vi "Voltage_Continuous_Output-Clear_data_when_stop.vi"() -> ()   [LabVIEW 2018]
doc: "This example demonstrates how to continuously re-generate analog output data from a buffer in your computer's memory.\n\nRefer to your device documentation for pinouts and hardware capabilities."
uses:
  <vilib>/Utility/error.llb/DialogType.ctl
  <vilib>/DAQmx/write.llb/DAQmx Write (Analog 1D Wfm NChan NSamp).vi
  <vilib>/DAQmx/create/channels.llb/DAQmx Create Channel (AO-Voltage-Basic).vi
  <vilib>/DAQmx/configure/timing.llb/DAQmx Timing (Sample Clock).vi
  <vilib>/DAQmx/miscellaneous.llb/DAQmx Fill In Error Info.vi
  <resource>/objmgr/daqmx.rc
  <vilib>/measure/NI_MABase.lvlib
panel:
  in  "Number of Samples":i32=1000
  in  "Output Array":T1(array[cluster])=[{"Waveform Type"=0, "Amplitude"=1.0, "Frequency"=10.0}] {"Frequency" format="%0.2p"; "Amplitude" format="%0.2p"; "Waveform Type" items=["Sine Wave", "Triangle Wave", "Square Wave", "Sawtooth Wave"]}
  in  "Stop":bool
  out "Waveform Graph":waveform(dbl)[](graph)=[{"t0"=timestamp(0 s since 1904-01-01), "dt"=0.001, "Y"=[]}]
  in  "Sample Rate":dbl=1000.0
  in  "Max Voltage":dbl=5.0
  in  "Min Voltage":dbl=-5.0
  in  "Physical Channel(s)":tag="Dev1/ao0"
  out "Actual Sample Rate":dbl=1000.0 format="%0.2f"
  # "Channel Settings"
  # "Output"
  # "Waveform Settings"
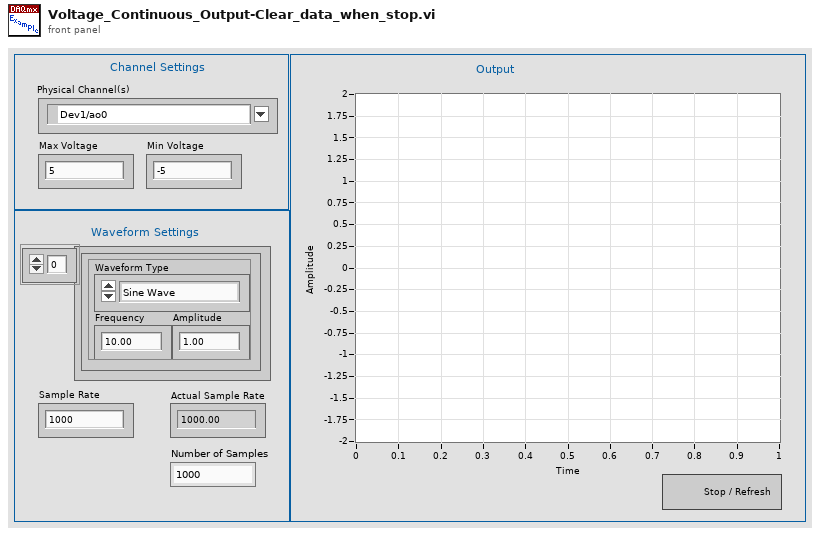
[diagram p1: front panel]
types:
  T1 = cluster{"Waveform Type":u16, "Amplitude":dbl, "Frequency":dbl}[]
  T2 = typedef "DialogType.ctl" = u16
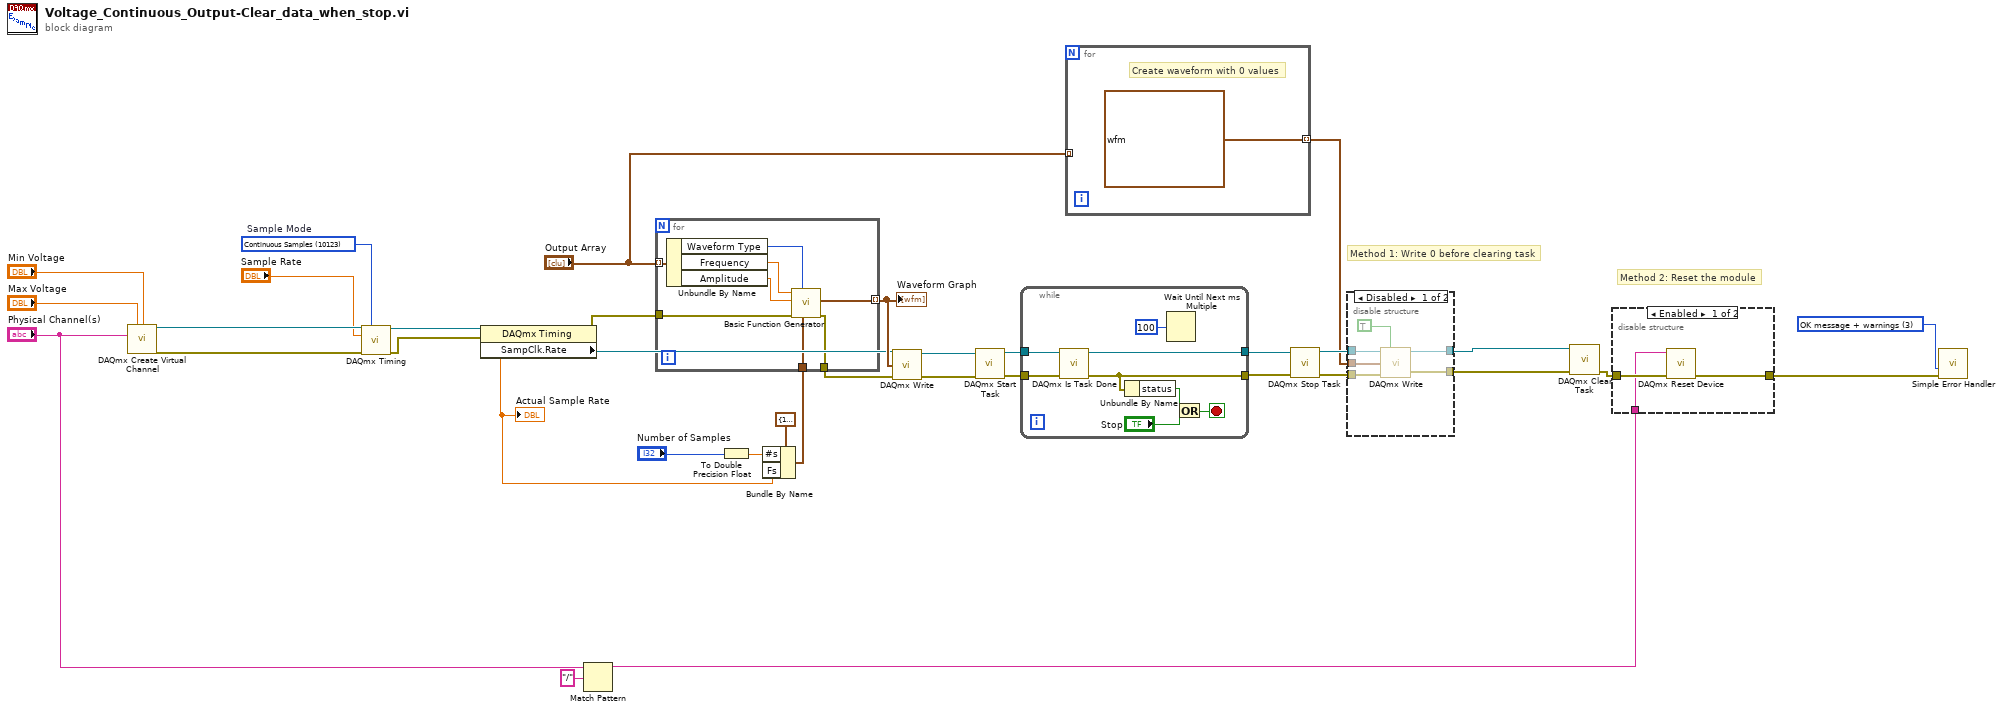
[diagram p0: block diagram]
diagram:
  w19 = T2 3 items=["no dialog", "OK message", "continue or stop message", "OK message + warnings", "continue/stop + warnings"] ("type of dialog (OK msg:1)")
  w33 = 10123 items=["Finite Samples"=10178, "Continuous Samples"=10123, "Hardware Timed Single Point"=12522]  # Sample Mode
  # "Method 2: Reset the module"
  # "Method 1: Write 0 before clearing task"
  n1 = call-poly <vilib>:"DAQmx Create Virtual Channel.vi"("maximum value"="Max Voltage", "minimum value"="Min Voltage", "physical channels"="Physical Channel(s)") -> ("task out"=w31:refnum<k21>, "error out"=w32:errorcluster)  [unwired: 11 in]
  n2 = call-poly <vilib>:"DAQmx Timing.vi"("task/channels in"=w31, "sample mode"=w33, "rate"="Sample Rate", "error in"=w32) -> ("task out"=w35:refnum<k21>, "error out"=w34:errorcluster)  [unwired: 10 in]
  n3 = property class="DAQmx Timing"(reference=w35, error in=w34) -> (reference out=w18:refnum<k21>, error out=w17:errorcluster, "SampClk.Rate"=w2:dbl)
  "Actual Sample Rate" <- w2
  n4 = Match Pattern(string="Physical Channel(s)", regular expression="/") -> (before substring=w12:string)  [unwired: 1 in, 3 out]
  n5 = To Double Precision Float(number="Number of Samples") -> (double precision float=w4:dbl)
  n6 = Bundle By Name(cluster=cluster{"Fs":dbl, "#s":dbl} {"Fs"=1000.0, "#s"=1000.0} ("sampling info"), "#s"=w4, "Fs"=w2) -> (w1:cluster{"Fs":dbl, "#s":dbl})
  n7 = for {
    tunnel: w17 -> [w43]
    tunnel: [w42] -> w23
    tunnel: "Output Array" -> [w41] mode=indexing
    tunnel: [w37] -> w22 mode=indexing
    tunnel: w1 -> [w36]
    n8 = Unbundle By Name(w41) -> ("Waveform Type"=w40:u16, "Frequency"=w39:dbl, "Amplitude"=w38:dbl)
    n9 = call <vilib>:"Basic Function Generator.vi"("sampling info"=w36, "signal type"=w40, "error in (no error)"=w43, "amplitude"=w38, "frequency"=w39) -> ("error out"=w42:errorcluster, "signal out"=w37:waveform(dbl))  [unwired: 4 in, 1 out]
  }
  "Waveform Graph" <- w22
  n10 = call-poly <vilib>:"DAQmx Write.vi"("task/channels in"=w18, "data"=w22, "error in"=w23) -> ("task out"=w25:refnum<k21>, "error out"=w24:errorcluster)  [unwired: 10 in, 1 out]
  n11 = call <vilib>:"DAQmx Start Task.vi"("task/channels in"=w25, "error in"=w24) -> ("task out"=w30:refnum<k21>, "error out"=w29:errorcluster)  [unwired: 12 in]
  n12 = while {
    tunnel: w30 -> [w51]
    tunnel: w29 -> [w50]
    tunnel: [w47] -> w20
    tunnel: [w48] -> w21
    stop <- w49 stop-if-true
    n13 = call <vilib>:"DAQmx Is Task Done.vi"("task/channels in"=w51, "error in"=w50) -> ("task out"=w48:refnum<k21>, "error out"=w47:errorcluster)  [unwired: 11 in, 1 out]
    n14 = Unbundle By Name(w47) -> ("status"=w46:bool)
    n15 = Wait Until Next ms Multiple(millisecond multiple=u32 100) -> ()  [unwired: 1 out]
    n16 = Or(x=w46, y="Stop") -> (x .or. y?=w49:bool)
  }
  n17 = for {
    tunnel: "Output Array" -> [_] mode=indexing
    tunnel: [waveform(dbl) {"t0"=timestamp(0 s since 1904-01-01), "dt"=1.0, "Y"=[0.0, 0.0, 0.0, 0.0, 0.0, 0.0, 0.0, 0.0, 0.0, 0.0, 0.0, 0.0, 0.0, 0.0]} ("signal out")] -> w8 mode=indexing
    # "Create waveform with 0 values"
  }
  n18 = call <vilib>:"DAQmx Stop Task.vi"("task/channels in"=w21, "error in"=w20) -> ("task out"=w9:refnum<k21>, "error out"=w10:errorcluster)  [unwired: 12 in]
  n19 = disable-structure "Diagram Disable Structure" shown="Disabled" {
    disable-tunnel: w10 -> [w57 w59]
    disable-tunnel: w9 -> [w56 w60]
    disable-tunnel: w8 -> [w55 _]
    disable-tunnel: [w54 w60] -> w7
    disable-tunnel: [w53 w59] -> w6
    frame Disabled {
      n20 = call-poly <vilib>:"DAQmx Write.vi"("task/channels in"=w56, "auto start"=TRUE, "data"=w55, "error in"=w57) -> ("task out"=w54:refnum<k21>, "error out"=w53:errorcluster)  [unwired: 9 in, 1 out]
    }
    frame Enabled {
    }
  }
  n21 = call <vilib>:"DAQmx Clear Task.vi"("task in"=w7, "error in"=w6) -> ("error out"=w15:errorcluster)  [unwired: 13 in]
  n22 = disable-structure "Diagram Disable Structure" shown="Enabled" {
    disable-tunnel: w15 -> [w63 w64]
    disable-tunnel: w12 -> [w62 _]
    disable-tunnel: [w61 w64] -> w11
    frame Enabled {
      n23 = call <vilib>:"DAQmx Reset Device.vi"("device in"=w62, "error in"=w63) -> ("error out"=w61:errorcluster)  [unwired: 13 in]
    }
    frame Disabled {
    }
  }
  n24 = call <vilib>:"Simple Error Handler.vi"("type of dialog (OK msg:1)"=w19, "error in (no error)"=w11) -> ()  [unwired: 3 in, 5 out]
